vi "xml anything to string.vi"() -> ()   [LabVIEW 2018]
uses:
  <vilib>/regexp/Match Regular Expression.xnode
panel:
  out "before match":string
  out "data string 3":string
  out "data string 2":string
  out "data string":string
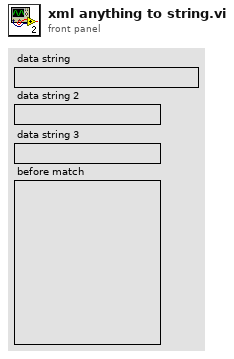
[diagram p1: front panel]
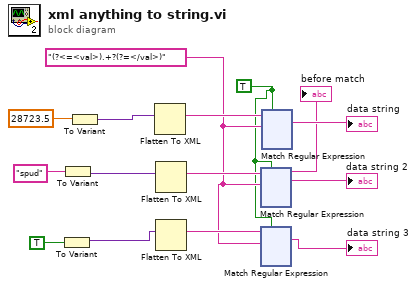
[diagram p0: block diagram]
diagram:
  w6 = "(?<=<val>).+?(?=</val>)" ("xml string")
  w1 = TRUE ("ignore case? (F)")
  n1 = To Variant(anything=TRUE) -> (Variant=w12:variant)
  n2 = To Variant(anything="spud") -> (Variant=w10:variant)
  n3 = To Variant(anything=28723.5) -> (Variant=w11:variant)
  n4 = Flatten To XML(anything=w11) -> (xml string=w7:string)
  n5 = Flatten To XML(anything=w10) -> (xml string=w8:string)
  n6 = Flatten To XML(anything=w12) -> (xml string=w9:string)
  n7 = xnode "Match Regular Expression"("input string"=w8, "regular expression"=w6, "ignore case? (F)"=w1) -> ("before match"=→"before match":string, "whole match"=→"data string 2":string)  [unwired: 3 in, 3 out]
  n8 = xnode "Match Regular Expression"("input string"=w9, "regular expression"=w6, "ignore case? (F)"=w1) -> ("whole match"=→"data string 3":string)  [unwired: 3 in, 4 out]
  n9 = xnode "Match Regular Expression"("input string"=w7, "regular expression"=w6, "ignore case? (F)"=w1) -> ("whole match"=→"data string":string)  [unwired: 3 in, 4 out]
